vi "Release.vi"(8 "error in (no error)":errorcluster, 11 "Module":T1) -> (0 "error out":errorcluster, 3 "Self":variant)   [LabVIEW 2022 SP3, in "Core.lvlib"]
uses:
  Core.lvlib
  Controls/Module.ctl
  Controls/Module Instance.ctl
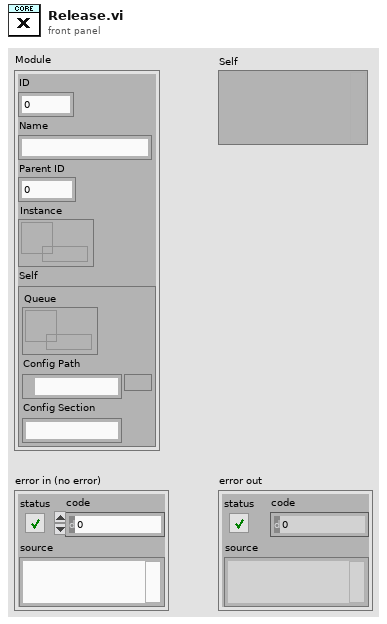
[diagram p1: front panel]
types:
  T1 = typedef "Core.lvlib/Module.ctl" = cluster{"ID":i32, "Name":string, "Parent ID":i32, "Instance":refnum<data-value>, "Self":T2}
  T2 = typedef "Core.lvlib/Module Instance.ctl" = cluster{"Queue":refnum<queue>, "Config Path":path, "Config Section":string}
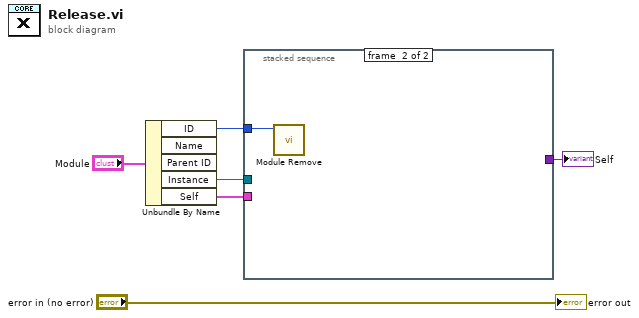
[diagram p0: block diagram]
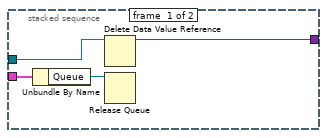
[diagram p2: hidden frame]
diagram:
  n1 = Unbundle By Name("Module") -> ("ID"=w3:i32, "Instance"=w2:refnum<data-value>, "Self"=w4:T2)  [unwired: 2 out]
  n2 = stacked-sequence {
    tunnel: w4 -> [w10 _]
    tunnel: w3 -> [_ w11]
    tunnel: w2 -> [w8 _]
    tunnel: [w7 _] -> w1
    frame #0 {
      n3 = Unbundle By Name(w10) -> ("Queue"=w9:refnum<queue>)
      n4 = Delete Data Value Reference(data value reference=w8) -> (data value=w7:variant)  [unwired: 1 in, 1 out]
      n5 = Release Queue(queue=w9) -> ()  [unwired: 2 in, 3 out]
    }
    frame #1 {
      n6 = call "Module Remove.vi"("ID"=w11) -> ()  [unwired: 9 in, 2 out]
    }
  }
  "Self" <- w1
  "error out" <- "error in (no error)"
